vi "VI Tree.vi"   [LabVIEW 2020, in "Keithley 622x.lvlib"]
doc: "This is the instrument driver for the Keithley 622x series of precision current sources. The VI Tree displays all the user-callable VIs of the instrument driver in an organized table."
uses:
  Keithley 622x.lvlib
panel:
  # "(c) 2014 FZD Keithley Instruments.  ALL RIGHTS RESERVED."
  # "SEE DIAGRAM\nFOR VI TREE."
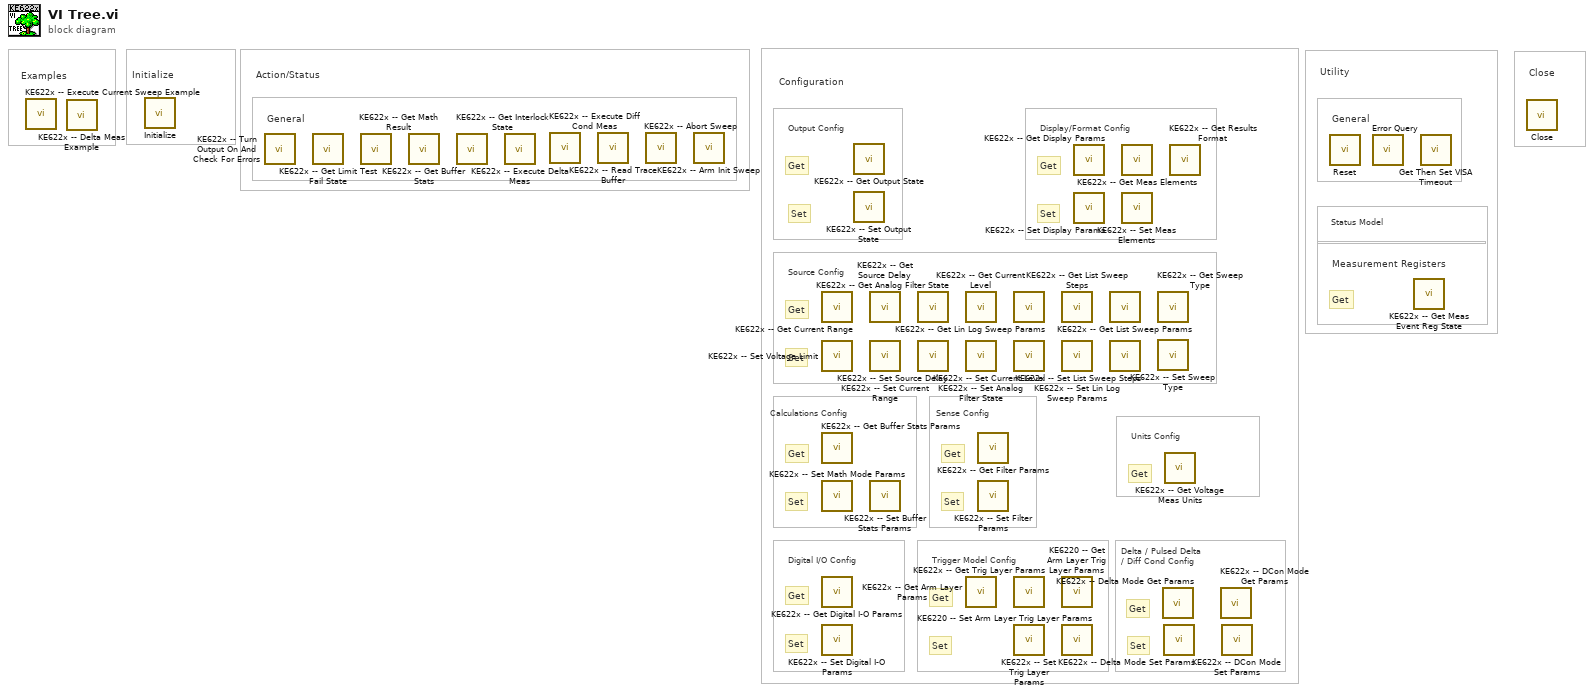
[diagram p0: block diagram]
diagram:
  # "Examples"
  # "Units Config"
  # "Get"
  # "Delta / Pulsed Delta \n/ Diff Cond Config"
  # "Get"
  # "Set"
  # "Trigger Model Config"
  # "Get"
  # "Set"
  # "Get"
  # "Set"
  # "Digital I/O Config"
  # "Get"
  # "Set"
  # "Sense Config"
  # "Calculations Config"
  # "Get"
  # "Set"
  # "General"
  # "General"
  # "Status Model"
  # "Source Config"
  # "Get"
  # "Set"
  # "Display/Format Config"
  # "Get"
  # "Set"
  # "Get"
  # "Set"
  # "Output Config"
  # "Get"
  # "Measurement Registers"
  # "Configuration"
  # "Utility"
  # "Action/Status"
  # "Close"
  # "Initialize"
  n1 = call "KE622x -- Execute Current Sweep Example.vi"() -> ()  [unwired: 1 in]
  n2 = call "KE622x -- Delta Meas Example.vi"() -> ()  [unwired: 1 in]
  n3 = call "Initialize.vi"() -> ()  [unwired: 14 in, 2 out]
  n4 = call "KE622x -- Turn Output On And Check For Errors.vi"() -> ()  [unwired: 12 in, 4 out]
  n5 = call "KE622x -- Get Limit Test Fail State.vi"() -> ()  [unwired: 13 in, 3 out]
  n6 = call "KE622x -- Get Math Result.vi"() -> ()  [unwired: 13 in, 3 out]
  n7 = call "KE622x -- Get Buffer Stats.vi"() -> ()  [unwired: 13 in, 3 out]
  n8 = call "KE622x -- Get Interlock State.vi"() -> ()  [unwired: 13 in, 3 out]
  n9 = call "KE622x -- Execute Delta Meas.vi"() -> ()  [unwired: 10 in, 6 out]
  n10 = call "KE622x -- Execute Diff Cond Meas.vi"() -> ()  [unwired: 10 in, 6 out]
  n11 = call "KE622x -- Read Trace Buffer.vi"() -> ()  [unwired: 13 in, 3 out]
  n12 = call "KE622x -- Abort Sweep.vi"() -> ()  [unwired: 14 in, 2 out]
  n13 = call "KE622x -- Arm Init Sweep.vi"() -> ()  [unwired: 14 in, 2 out]
  n14 = call "KE622x -- Get Current Range.vi"() -> ()  [unwired: 13 in, 3 out]
  n15 = call "KE622x -- Set Voltage Limit.vi"() -> ()  [unwired: 14 in, 2 out]
  n16 = call "KE622x -- Get Buffer Stats Params.vi"() -> ()  [unwired: 13 in, 3 out]
  n17 = call "KE622x -- Set Math Mode Params.vi"() -> ()  [unwired: 13 in, 3 out]
  n18 = call "KE622x -- Get Digital I-O Params.vi"() -> ()  [unwired: 13 in, 3 out]
  n19 = call "KE622x -- Set Digital I-O Params.vi"() -> ()  [unwired: 14 in, 2 out]
  n20 = call "KE622x -- Get Output State.vi"() -> ()  [unwired: 13 in, 3 out]
  n21 = call "KE622x -- Set Output State.vi"() -> ()  [unwired: 14 in, 2 out]
  n22 = call "KE622x -- Get Source Delay.vi"() -> ()  [unwired: 13 in, 3 out]
  n23 = call "KE622x -- Set Current Range.vi"() -> ()  [unwired: 13 in, 3 out]
  n24 = call "KE622x -- Set Buffer Stats Params.vi"() -> ()  [unwired: 14 in, 2 out]
  n25 = call "KE622x -- Get Analog Filter State.vi"() -> ()  [unwired: 13 in, 3 out]
  n26 = call "KE622x -- Set Source Delay.vi"() -> ()  [unwired: 13 in, 3 out]
  n27 = call "KE622x -- Get Current Level.vi"() -> ()  [unwired: 13 in, 3 out]
  n28 = call "KE622x -- Set Analog Filter State.vi"() -> ()  [unwired: 14 in, 2 out]
  n29 = call <instrlib>:"KE622x -- Get Arm Layer Params.vi"() -> ()  [unwired: 13 in, 3 out]
  n30 = call "KE622x -- Get Filter Params.vi"() -> ()  [unwired: 13 in, 3 out]
  n31 = call "KE622x -- Set Filter Params.vi"() -> ()  [unwired: 13 in, 3 out]
  n32 = call "KE622x -- Get Lin Log Sweep Params.vi"() -> ()  [unwired: 13 in, 3 out]
  n33 = call "KE622x -- Set Current Level.vi"() -> ()  [unwired: 13 in, 3 out]
  n34 = call "KE622x -- Get Trig Layer Params.vi"() -> ()  [unwired: 13 in, 3 out]
  n35 = call "KE622x -- Set Trig Layer Params.vi"() -> ()  [unwired: 13 in, 3 out]
  n36 = call <instrlib>:"KE622x -- Get List Sweep Steps.vi"() -> ()  [unwired: 12 in, 4 out]
  n37 = call "KE622x -- Set Lin Log Sweep Params.vi"() -> ()  [unwired: 13 in, 3 out]
  n38 = call "KE6220 -- Get Arm Layer Trig Layer Params.vi"() -> ()  [unwired: 13 in, 3 out]
  n39 = call "KE6220 -- Set Arm Layer Trig Layer Params.vi"() -> ()  [unwired: 13 in, 3 out]
  n40 = call "KE622x -- Get Display Params.vi"() -> ()  [unwired: 13 in, 3 out]
  n41 = call "KE622x -- Set Display Params.vi"() -> ()  [unwired: 14 in, 2 out]
  n42 = call <instrlib>:"KE622x -- Get List Sweep Params.vi"() -> ()  [unwired: 13 in, 3 out]
  n43 = call <instrlib>:"KE622x -- Set List Sweep Steps.vi"() -> ()  [unwired: 13 in, 3 out]
  n44 = call "KE622x -- Get Meas Elements.vi"() -> ()  [unwired: 13 in, 3 out]
  n45 = call "KE622x -- Set Meas Elements.vi"() -> ()  [unwired: 14 in, 2 out]
  n46 = call "KE622x -- Get Sweep Type.vi"() -> ()  [unwired: 13 in, 3 out]
  n47 = call "KE622x -- Set Sweep Type.vi"() -> ()  [unwired: 14 in, 2 out]
  n48 = call "KE622x -- Delta Mode Get Params.vi"() -> ()  [unwired: 13 in, 3 out]
  n49 = call "KE622x -- Delta Mode Set Params.vi"() -> ()  [unwired: 13 in, 3 out]
  n50 = call "KE622x -- Get Voltage Meas Units.vi"() -> ()  [unwired: 13 in, 3 out]
  n51 = call "KE622x -- Get Results Format.vi"() -> ()  [unwired: 13 in, 3 out]
  n52 = call "KE622x -- DCon Mode Get Params.vi"() -> ()  [unwired: 13 in, 3 out]
  n53 = call "KE622x -- DCon Mode Set Params.vi"() -> ()  [unwired: 11 in, 5 out]
  n54 = call "Reset.vi"() -> ()  [unwired: 14 in, 2 out]
  n55 = call "Error Query.vi"() -> ()  [unwired: 12 in, 4 out]
  n56 = call "KE622x -- Get Meas Event Reg State.vi"() -> ()  [unwired: 13 in, 3 out]
  n57 = call "Get Then Set VISA Timeout.vi"() -> ()  [unwired: 12 in, 4 out]
  n58 = call "Close.vi"() -> ()  [unwired: 15 in, 1 out]
